vi "solar_tcp Config.vi"(5 "Action (Read)":enum8{"Read", "Write"}(ring), 7 "Section (\"\" = Use Filename)":string, 8 "error in (no error)":errorcluster, 9 "Key Prefix ('tcp.')":string="tcp.", 10 "Config in":T1={"TCPServer"=enum."SERVER", "ServerPort"=0, "IPAddress"="", "ClientPort"=0, "HdrSizeBytes"=4, "HdrLenSubtractBytes"=4, "HdrLenOffsetBits"=0, "HdrLenSizeBits"=32}, 11 "Path in":path) -> (0 "error out":errorcluster, 2 "Config out":T1, 3 "Path out":path)   [LabVIEW 2018]
doc: "This loads TCP setting from a configuration file. The default key prefix is 'tcp.'.\nvi_tree:4-4"
uses:
  cfg/solar_cfg Read File (Var).vi
  cfg/solar_cfg Write File (Var).vi
  solar_tcp_ctl Config.ctl
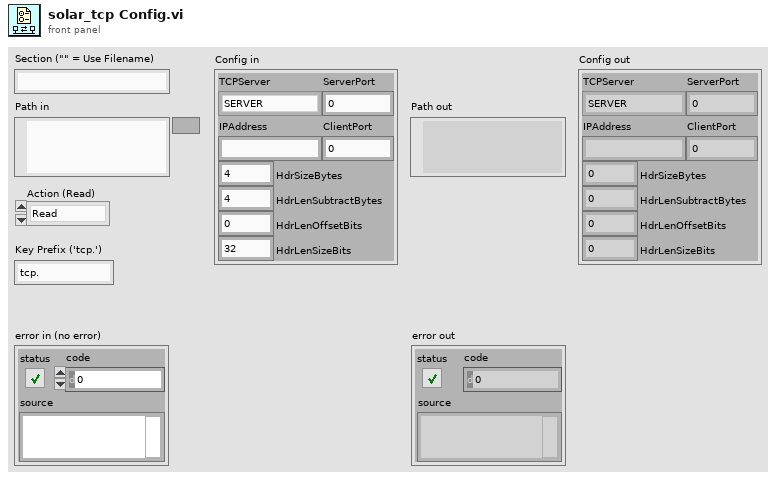
[diagram p1: front panel]
types:
  T1 = typedef "solar_tcp_ctl Config.ctl" = cluster{"TCPServer":enum8{"SERVER", "CLIENT"}, "ServerPort":u16, "IPAddress":string, "ClientPort":u16, "HdrSizeBytes":i32, "HdrLenSubtractBytes":i32, "HdrLenOffsetBits":i32, "HdrLenSizeBits":i32}
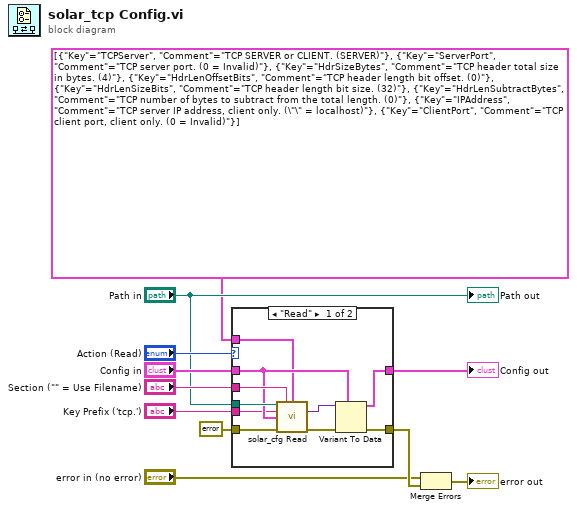
[diagram p0: block diagram]
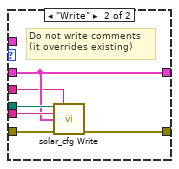
[diagram p2: hidden frame]
diagram:
  n1 = case shown="\"Read\"" "Action (Read)" {
    tunnel: errorcluster {"status"=FALSE, "code"=0, "source"=""} ("error in (no error)") -> [w21 w27]
    tunnel: "Path in" -> [w20 w25]
    tunnel: "Section (\"\" = Use Filename)" -> [w19 w22]
    tunnel: "Config in" -> [w16 w23]
    tunnel: [w15 w26] -> w11
    tunnel: "Key Prefix ('tcp.')" -> [w14 w24]
    tunnel: [w13 w23] -> w7
    tunnel: cluster{"Key":string, "Comment":string}[] [{"Key"="TCPServer", "Comment"="TCP SERVER or CLIENT. (SERVER)"}, {"Key"="ServerPort", "Comment"="TCP server port. (0 = Invalid)"}, {"Key"="HdrSizeBytes", "Comment"="TCP header total size in bytes. (4)"}, {"Key"="HdrLenOffsetBits", "Comment"="TCP header length bit offset. (0)"}, {"Key"="HdrLenSizeBits", "Comment"="TCP header length bit size. (32)"}, {"Key"="HdrLenSubtractBytes", "Comment"="TCP number of bytes to subtract from the total length. (0)"}, {"Key"="IPAddress", "Comment"="TCP server IP address, client only. (\"\" = localhost)"}, {"Key"="ClientPort", "Comment"="TCP client port, client only. (0 = Invalid)"}] ("Comments (Key,Comment)") -> [w12 _]
    frame "Read" {
      n2 = call-poly "solar_cfg Read.vi"("Config Path (*.ini)"=w20, "Section (\"\" = Use Filename)"=w19, "Comments (Key,Comment)"=w12, "Key_Prefix (\"\")"=w14, "Variant in"=w16, "error in (no error)"=w21) -> ("Variant out"=w17:variant, "error out"=w18:errorcluster)  [unwired: 6 in, 2 out]
      n3 = Variant To Data(error in=w18, type=w16, Variant=w17) -> (data=w13:T1, error out=w15:errorcluster)
    }
    frame "Write" {
      # "Do not write comments\n(it overrides existing)"
      n4 = call-poly "solar_cfg Write.vi"("Config Path (*.ini)"=w25, "Section (\"\" = Use Filename)"=w22, "Key_Prefix (\"\")"=w24, "Variant"=w23, "error in (no error)"=w27) -> ("error out"=w26:errorcluster)  [unwired: 8 in, 2 out]
    }
  }
  "Config out" <- w7
  n5 = Merge Errors("error in (no error)", w11) -> (→"error out":errorcluster)
  "Path out" <- "Path in"
